vi "Test_OpenCloseCommunicator.vi"(8 "error in (no error)":errorcluster) -> (0 "error out":errorcluster)   [LabVIEW 2023, in "horiba.test.lvlib"]
uses:
  Classes/Communicator/Communicator.lvclass
  <vilib>/addons/_JKI Toolkits/Caraya/classes/Assert/Assert Not Error.vi
  horiba.test.lvlib
  <vilib>/addons/_JKI Toolkits/Caraya/classes/Test/Test.lvclass
  <vilib>/addons/_JKI Toolkits/Caraya/classes/Assert/Assert.lvclass
panel:
  # "Connector Pane"
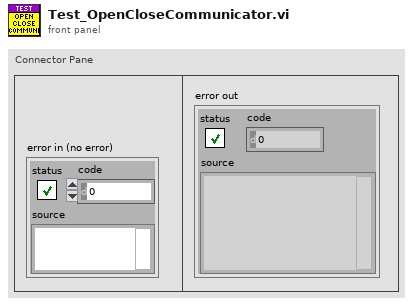
[diagram p1: front panel]
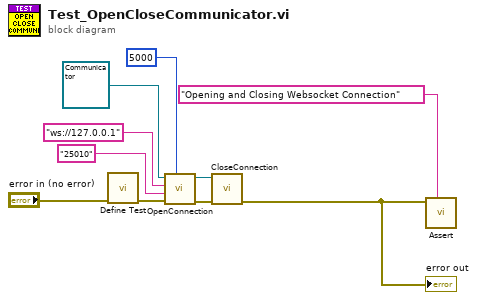
[diagram p0: block diagram]
diagram:
  n1 = call <vilib>:"Define Test.vi"("error in (no error)"="error in (no error)") -> ("error out"=w7:errorcluster)  [unwired: 9 in, 1 out]
  n2 = call-dynamic "OpenConnection.vi"("timeout opening [ms]"=5000, "error in (no error)"=w7, "WS Server Port"="25010", "WS Server IP"="ws://127.0.0.1", "Communicator in"=refnum<class "Communicator.lvclass"> refnum) -> ("error out"=w4:errorcluster, "Communicator out"=w5:refnum<class "Communicator.lvclass">)  [unwired: 4 in, 1 out]
  n3 = call-dynamic "CloseConnection.vi"("error in (no error)"=w4, "Communicator in"=w5) -> ("error out"=w3:errorcluster)  [unwired: 8 in, 1 out]
  "error out" <- w3
  n4 = call-poly <vilib>:"Assert.vi"("Label"="Opening and Closing Websocket Connection", "Not Error?"=w3) -> ()  [unwired: 8 in, 2 out]
